vi "Sub-dealwith.vi"(9 "Angle (Pixel) 2":dbl, 10 "Center 3":cluster{"X":sgl, "Y":sgl}, 11 "Center 2":cluster{"X":sgl, "Y":sgl}) -> (0 "Y":string, 1 "X":string, 2 "5.4":string, 3 "45.03":string, 4 "最终角度":string, 5 "Distance":string)   [LabVIEW 2015]
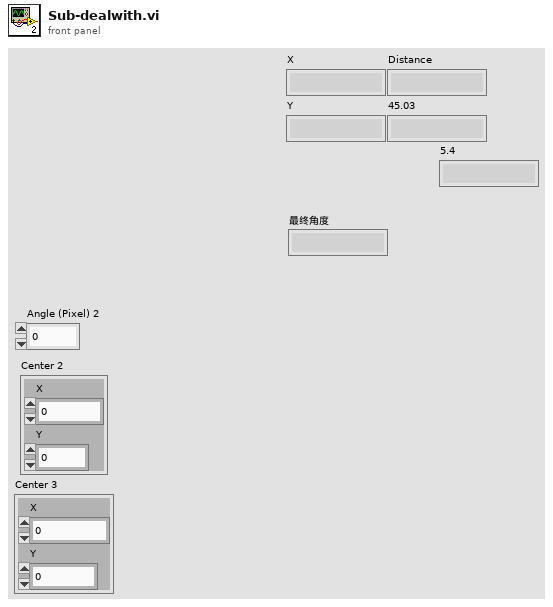
[diagram p1: front panel]
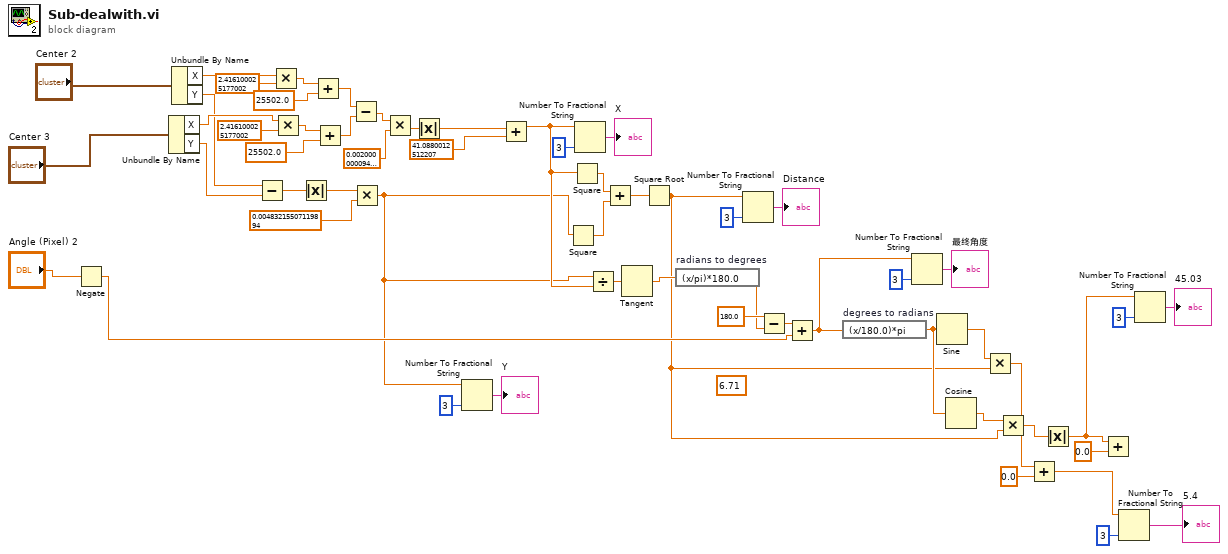
[diagram p0: block diagram]
diagram:
  (unwired) 6.71
  n1 = Negate(x="Angle (Pixel) 2") -> (-x=w19:dbl)
  n2 = Unbundle By Name("Center 3") -> ("X"=w50:sgl, "Y"=w41:sgl)
  n3 = Unbundle By Name("Center 2") -> ("X"=w57:sgl, "Y"=w42:sgl)
  n4 = Subtract(x=w42, y=w41) -> (x-y=w37:sgl)
  n5 = Multiply(x=w57, y=sgl 2.4161) -> (x*y=w55:sgl)
  n6 = Multiply(x=w50, y=sgl 2.4161) -> (x*y=w52:sgl)
  n7 = Absolute Value(x=w37) -> (abs(x)=w36:sgl)
  n8 = Add(x=w55, y=sgl 25502.0) -> (x+y=w49:sgl)
  n9 = Add(x=w52, y=sgl 25502.0) -> (x+y=w48:sgl)
  n10 = Subtract(x=w49, y=w48) -> (x-y=w46:sgl)
  n11 = Multiply(x=w36, y=sgl 0.004832155) -> (x*y=w14:sgl)
  n12 = Multiply(x=w46, y=sgl 0.002) -> (x*y=w44:sgl)
  n13 = Absolute Value(x=w44) -> (abs(x)=w43:sgl)
  n14 = Number To Fractional String(number=w14, precision (6)=i16 3 ("精度(6)")) -> (F-format string=→"Y":string)  [unwired: 2 in]
  n15 = Add(x=w43, y=sgl 41.088) -> (x+y=w18:sgl)
  n16 = Square(x=w14) -> (x^2=w39:sgl)
  n17 = Square(x=w18) -> (x^2=w40:sgl)
  n18 = Number To Fractional String(number=w18, precision (6)=i16 3 ("精度(6)")) -> (F-format string=→"X":string)  [unwired: 2 in]
  n19 = Divide(x=w14, y=w18) -> (x/y=w35:sgl)
  n20 = Add(x=w40, y=w39) -> (x+y=w38:sgl)
  n21 = Tangent(1:w35) -> (0:w34:sgl)
  n22 = Square Root(x=w38) -> (sqrt(x)=w11:sgl)
  n23 = expression code="(x/pi)*180.0" "radians to degrees"(w34) -> (w29:sgl)
  n24 = Number To Fractional String(number=w11, precision (6)=i16 3 ("精度(6)")) -> (F-format string=→"Distance":string)  [unwired: 2 in]
  n25 = Subtract(x=180.0, y=w29) -> (x-y=w28:dbl)
  n26 = Add(x=w28, y=w19) -> (x+y=w2:dbl)
  n27 = expression code="(x/180.0)*pi" "degrees to radians"(w2) -> (w32:dbl)
  n28 = Number To Fractional String(number=w2, precision (6)=i16 3 ("精度(6)")) -> (F-format string=→"最终角度":string)  [unwired: 2 in]
  n29 = Sine(x=w32) -> (sin(x)=w33:dbl)
  n30 = Cosine(x=w32) -> (cos(x)=w31:dbl)
  n31 = Multiply(x=w33, y=w11) -> (x*y=w26:dbl)
  n32 = Multiply(x=w31, y=w11) -> (x*y=w27:dbl)
  n33 = Add(x=w26, y=0.0) -> (x+y=w4:dbl)
  n34 = Absolute Value(x=w27) -> (abs(x)=w8:dbl)
  n35 = Add(x=w8, y=0.0) -> ()  [unwired: 1 out]
  n36 = Number To Fractional String(number=w4, precision (6)=i16 3 ("精度(6)")) -> (F-format string=→"5.4":string)  [unwired: 2 in]
  n37 = Number To Fractional String(number=w8, precision (6)=i16 3 ("精度(6)")) -> (F-format string=→"45.03":string)  [unwired: 2 in]
